vi "BMU参数读取-Auto.vi"(7 "Socket":dbl, 8 "CAN端口":u16(ring), 9 "设备索引号":u16(ring), 10 "CAN卡类型":u32(ring)=21, 11 "从板号":u8=1) -> (3 "成功?":bool)   [LabVIEW 2013] (continued)
                  n499 = local read "设备索引号"() -> (w673:u16)
                  n500 = local read "CAN卡类型"() -> (w674:u32)
                  n501 = Increment(x=w670) -> (x+1=w667:dbl)
                  n502 = local read "CAN端口"() -> (w672:u16)
                  n503 = Reshape Array(w671, w667) -> (w669:dbl[])
                  n504 = stacked-sequence {
                    tunnel: w674 -> [_ w682]
                    tunnel: w673 -> [_ w681]
                    tunnel: w672 -> [_ w680]
                    tunnel: w669 -> [_ w679]
                    tunnel: w668 -> [_ w678]
                    tunnel: w666 -> [_ w677]
                    tunnel: w665 -> [_ w676]
                    frame #0 {
                    }
                    frame #1 {
                      n505 = call "多帧发送机制(EV05).vi"("can卡类型"=w682, "设备索引号"=w681, "CAN端口"=w680, "命令"=w676, "板号"=w678, "命令序号"=w677, "输入数据"=w679) -> ("错误输出"=w675:errorcluster)  [unwired: 2 in, 10 out]
                      n506 = call <vilib>:"Clear Errors.vi"("error in (no error)"=w675) -> ()  [unwired: 6 in, 1 out]
                    }
                  }
                }
                frame #3 {
                  n507 = while {
                    tunnel: [w685] -> w683
                    i -> [w690]
                    stop <- w687 stop-if-true
                    n508 = local read "强制终止读写标记"() -> (w684:bool)
                    n509 = global read "EV05全局变量1.vi" "读取超时"() -> (w685:bool)
                    n510 = Greater Or Equal?(x=w690, y=30) -> (x >= y?=w688:bool)
                    n511 = Wait Until Next ms Multiple(millisecond multiple=u32 100 ("毫秒倍数")) -> ()  [unwired: 1 out]
                    n512 = Compound Arithmetic op=OR(w684, w685, w688) -> (w687:bool)
                  }
                }
                frame #4 {
                  n513 = call <vilib>:"Unset Busy.vi"() -> ()  [unwired: 2 in, 10 out]
                  n514 = case shown="假" w692 {
                    tunnel: w691 -> [w693 _]
                    frame False {
                      n515 = control-ref of="结果"() -> (w697:refnum<vi>)
                      n516 = Concatenate Strings(w693, "       写入失败" ("字符串")) -> (w696:string)
                      n517 = Build Array(w696) -> (w695:string[])
                      n518 = call "表格编辑.vi"("新元素/子数组"=w695, "活动单元格:单元格背景色"=u32 16740749, "MCListbox引用句柄"=w697) -> ()  [unwired: 9 out]
                    }
                    frame True {
                    }
                  }
                }
                frame #5 {
                  n519 = Increment(x=w703) -> (x+1=w699:i32)
                  n520 = Equal?(x=w704, y=w699) -> (x = y?=w702:bool)
                  n521 = And(x=w701, y=w702) -> (x .and. y?=w700:bool)
                  n522 = case shown="真" w700 {
                    frame False {
                    }
                    frame True {
                      n523 = control-ref of="结果"() -> (w708:refnum<vi>)
                      n524 = Concatenate Strings("写入完成" ("字符串")) -> (w707:string)
                      n525 = Build Array(w707) -> (w706:string[])
                      n526 = call "表格编辑.vi"("新元素/子数组"=w706, "活动单元格:单元格背景色"=u32 21937, "MCListbox引用句柄"=w708) -> ()  [unwired: 9 out]
                    }
                  }
                }
              }
            }
            n527 = local read "强制终止读写标记"() -> (w601:bool)
            n528 = Or(x=w599, y=w601) -> (x .or. y?=w600:bool)
          }
          n529 = stacked-sequence {
            tunnel: w591 -> [_]
            frame #0 {
              n530 = call <vilib>:"Unset Busy.vi"() -> ()  [unwired: 2 in, 10 out]
              n531 = local write "强制终止读写标记"(FALSE ("强制停止")) -> ()
            }
          }
        }
        frame "单个读取" {
          n532 = stacked-sequence {
            tunnel: [w741] -> w739
            frame #0 {
              n533 = local read "主从选择"() -> (w742:enum32{"主板", "从板"})
              n534 = case shown="\"主板\", 默认" w742 {
                tunnel: [w755 w838] -> w744
                tunnel: [w754 w839] -> w749
                tunnel: [0 ("从板号") w835] -> w748
                tunnel: [0 ("板号") u8 0 ("板号")] -> w747
                tunnel: [w750 w834] -> w745
                frame "主板", Default {
                  n535 = local read "主板选项"() -> (w751:string)
                  n536 = case shown="\"二维码\"" w751 {
                    tunnel: [_ u8[] [1, 2, 3, 4, 5, 6, 13, 8, 7, 9, 10, 11, 12] u8[] [1] u8[] [1] u8[] [1] u8[] [2] u8[] [3] u8[] [4] u8[] [5] u8[] [6] u8[] [13] u8[] [7] u8[] [8] u8[] [9] u8[] [10] u8[] [14] u8[] [11] u8[] [12] u8[] [2] u8[] [3] u8[] [1] u8[] [2] u8[] [1] u8[] [2] u8[] [3] u8[] [4] u8[] [1, 2, 3, 4]] -> w755
                    tunnel: [_ u8 128 ("命令") u8 129 ("命令") u8 128 ("命令") u8 140 ("命令") u8 128 ("命令") u8 128 ("命令") u8 128 ("命令") u8 128 ("命令") u8 128 ("命令") u8 128 ("命令") u8 128 ("命令") u8 128 ("命令") u8 128 ("命令") u8 128 ("命令") u8 128 ("命令") u8 128 ("命令") u8 128 ("命令") u8 129 ("命令") u8 129 ("命令") u8 130 ("命令") u8 130 ("命令") u8 132 ("命令") u8 132 ("命令") u8 132 ("命令") u8 132 ("命令") u8 132 ("命令")] -> w754
                    tunnel: [_ string[] ["产品编号", "电压个数", "通道电压数", "电压起始值", "温度个数", "温度起始值", "保险位置", "电池额定实际容量", "SOC", "配置文件版本", "参数修改记录", "车牌号", "SOH"] string[] ["一级故障阀值"] string[] ["产品编号"] string[] ["读二维码"] string[] ["电压个数"] string[] ["通道电压数"] string[] ["电压起始值"] string[] ["温度个数"] string[] ["温度起始值"] string[] ["保险位置"] string[] ["SOC"] string[] ["电池额定实际容量"] string[] ["配置文件版本"] string[] ["参数修改记录"] string[] ["校正时钟"] string[] ["车牌号"] string[] ["SOH"] string[] ["二级故障阀值"] string[] ["三级故障阀值"] string[] ["加热控制参数"] string[] ["充电控制参数"] string[] ["电池信息1"] string[] ["电池包组号"] string[] ["充放电安时"] string[] ["电池充放电次数"] string[] ["电池信息1", "电池包组号", "充放电安时", "电池充放电次数"]] -> w750
                    frame "假", Default {
                    }
                    frame "项目信息" {
                    }
                    frame "SOC过低", "SOC过高", "SOH过低", "充电电流过高", "单体电压过低", "单体电压过高", "单组电压不均衡", "单组温度不均衡", "放电电流过高", "极柱温度过高", "内阻过大", "温度过低", "温度过高", "一级故障阀值", "整组电压不均衡", "整组温度不均衡", "总电压过低", "总电压过高" {
                    }
                    frame "产品编号" {
                    }
                    frame "二维码" {
                    }
                    frame "电压个数" {
                    }
                    frame "通道电压数" {
                    }
                    frame "电压起始值" {
                    }
                    frame "温度个数" {
                    }
                    frame "温度起始值" {
                    }
                    frame "保险位置" {
                    }
                    frame "SOC" {
                    }
                    frame "电池额定实际容量" {
                    }
                    frame "配置文件版本" {
                    }
                    frame "参数修改记录" {
                    }
                    frame "校正时钟" {
                    }
                    frame "车牌号" {
                    }
                    frame "SOH" {
                    }
                    frame "SOC过低(2)", "SOC过高(2)", "SOH过低(2)", "充电电流过高(2)", "单体电压过低(2)", "单体电压过高(2)", "单组电压不均衡(2)", "单组温度不均衡(2)", "二级故障阀值", "放电电流过高(2)", "极柱温度过高(2)", "内阻过大(2)", "温度过低(2)", "温度过高(2)", "整组电压不均衡(2)", "整组温度不均衡(2)", "总电压过低(2)", "总电压过高(2)" {
                    }
                    frame "SOC过低(3)", "SOC过高(3)", "SOH过低(3)", "充电电流过高(3)", "单体电压过低(3)", "单体电压过高(3)", "单组电压不均衡(3)", "单组温度不均衡(3)", "放电电流过高(3)", "极柱温度过高(3)", "内阻过大(3)", "三级故障阀值", "温度过低(3)", "温度过高(3)", "整组电压不均衡(3)", "整组温度不均衡(3)", "总电压过低(3)", "总电压过高(3)" {
                    }
                    frame "风机关闭温差", "风机关闭温度", "风机开启温差", "风机开启温度", "加热关闭温差", "加热关闭温度", "加热开启温度", "加热控制参数" {
                    }
                    frame "充电控制参数", "电流步长", "最大允许充电电流", "最大允许充电温度", "最大允许单体电压", "最大允许总电压", "最小允许充电电流", "最小允许充电温度", "最小允许单体电压" {
                    }
                    frame "电池信息1" {
                    }
                    frame "电池包组号" {
                    }
                    frame "充放电安时" {
                    }
                    frame "电池充放电次数" {
                    }
                    frame "电池信息" {
                    }
                  }
                }
                frame "从板" {
                  n537 = local read "从板选项"() -> (w836:string)
                  n538 = case shown="\"二维码\"" w836 {
                    tunnel: [_ u8 0 ("命令") u8 10 ("命令") u8 0 ("命令") u8 0 ("命令") u8 0 ("命令") u8 0 ("命令") u8 0 ("命令") u8 0 ("命令") u8 2 ("命令") u8 2 ("命令") u8 2 ("命令") u8 3 ("命令") u8 6 ("命令") u8 6 ("命令") u8 6 ("命令") u8 3 ("命令") u8 3 ("命令") u8 3 ("命令") u8 3 ("命令") u8 3 ("命令") u8 3 ("命令") u8 3 ("命令")] -> w839
                    tunnel: [_ u8[] [6] u8[] [1] u8[] [6, 1, 2, 3, 4, 5] u8[] [1] u8[] [2] u8[] [3] u8[] [4] u8[] [5] u8[] [1] u8[] [2] u8[] [3] u8[] [1, 2, 3, 4, 5, 6, 7] u8[] [1, 2] u8[] [2] u8[] [1] u8[] [1] u8[] [2] u8[] [3] u8[] [4] u8[] [5] u8[] [6] u8[] [7]] -> w838
                    tunnel: [_ string[] ["从板号"] string[] ["读二维码"] string[] ["从板号", "电压起始值", "通道电压个数", "保险位置", "温度起始值", "加热控制参数"] string[] ["电压起始值"] string[] ["通道电压节数"] string[] ["保险位置"] string[] ["温度起始值"] string[] ["加热控制参数"] string[] ["一级故障阀值"] string[] ["二级故障阀值"] string[] ["三级故障阀值"] string[] ["电池包信息1", "电池包序号", "充放电安时", "充电次数时间", "SOC", "车牌号", "充电参数"] string[] ["均衡阀值", "充电结束电压"] string[] ["充电结束电压"] string[] ["均衡阀值"] string[] ["电池包信息1"] string[] ["电池包序号"] string[] ["充放电安时"] string[] ["充电次数时间"] string[] ["SOC"] string[] ["车牌号"] string[] ["充电参数"]] -> w834
                    frame "假", Default {
                    }
                    frame "从板号" {
                    }
                    frame "二维码" {
                    }
                    frame "从板信息" {
                    }
                    frame "电压个数" {
                    }
                    frame "通道电压节数" {
                    }
                    frame "保险位置" {
                    }
                    frame "温度个数" {
                    }
                    frame "风机关闭温差", "风机关闭温度", "风机开启温差", "风机开启温度", "加热关闭温差", "加热关闭温度", "加热开启温度", "加热控制参数" {
                    }
                    frame "SOC过低", "电压不均衡", "电压过低", "电压过高", "温度不均衡", "温度过低", "温度过高", "一级故障阀值" {
                    }
                    frame "SOC过低(2)", "电压不均衡(2)", "电压过低(2)", "电压过高(2)", "二级故障阀值", "温度不均衡(2)", "温度过低(2)", "温度过高(2)" {
                    }
                    frame "SOC过低(3)", "电压不均衡(3)", "电压过低(3)", "电压过高(3)", "三级故障阀值", "温度不均衡(3)", "温度过低(3)", "温度过高(3)" {
                    }
                    frame "快换参数" {
                    }
                    frame "均衡参数" {
                    }
                    frame "充电结束电压" {
                    }
                    frame "均衡阀值" {
                    }
                    frame "电池包信息1" {
                    }
                    frame "电池包序号" {
                    }
                    frame "充放电安时" {
                    }
                    frame "充电次数时间" {
                    }
                    frame "SOC" {
                    }
                    frame "车牌号" {
                    }
                    frame "充电参数" {
                    }
                  }
                  n539 = local read "从板号"() -> (w835:u8)
                }
              }
              n540 = Build Array(w747) -> (w746:i32[])
              n541 = local write "命令"(w749) -> ()
              n542 = Array Size(array=w744) -> (size(s)=w743:i32)
              n543 = for {
                tunnel: w744 -> [w914] mode=indexing
                tunnel: w749 -> [w913]
                tunnel: w748 -> [w912]
                tunnel: w746 -> [w911]
                tunnel: w745 -> [w910] mode=indexing
                tunnel: w743 -> [w909]
                tunnel: w742 -> [w907]
                tunnel: [w906] -> w741
                i -> [w908]
                n544 = while {
                  tunnel: w914 -> [w923]
                  tunnel: w913 -> [w922]
                  tunnel: w912 -> [w921]
                  tunnel: w911 -> [w920]
                  tunnel: w910 -> [w919]
                  tunnel: w909 -> [w918]
                  tunnel: w908 -> [w917]
                  tunnel: w907 -> [w916]
                  tunnel: [w915] -> w906
                  stop <- w915 stop-if-true
                  n545 = stacked-sequence {
                    seq-local: [_ _ _ _ w1073 _ _] -> [_ _ _ _ _ w1082 _]
                    tunnel: w923 -> [_ _ _ w1061 _ _ _]
                    tunnel: w922 -> [_ _ _ w1060 _ _ _]
                    tunnel: w921 -> [_ _ _ w1059 _ _ _]
                    tunnel: w920 -> [_ _ _ w1058 _ _ _]
                    tunnel: [_ _ _ _ w1074 _ _] -> w915
                    tunnel: w919 -> [w925 _ _ _ _ w1083 _]
                    tunnel: w918 -> [_ _ _ _ _ _ w1093]
                    tunnel: w917 -> [_ _ _ _ _ _ w1092]
                    tunnel: w916 -> [w924 _ _ _ _ _ _]
                    frame #0 {
                      n546 = case shown="\"从板\"" w924 {
                        tunnel: w925 -> [w926 w1018]
                        frame "主板", Default {
                          n547 = case shown="\"读二维码\"" w926 {
                            frame "假", Default {
                            }
                            frame "产品编号" {
                              n548 = control-ref of="产品编号"() -> (w928:refnum<vi>)
                              n549 = property class="Str"(reference=w928, "Value"="") -> ()  [unwired: 1 in, 2 out]
                            }
                            frame "读二维码" {
                              n550 = local write "二维码信息"("" ("二维码信息")) -> ()
                            }
                            frame "电压个数" {
                              n551 = local read "从板个数"() -> (w930:dbl)
                              n552 = control-ref of="项目信息"() -> (w934:refnum<vi>)
                              n553 = for {
                                N: w930 -> [_]
                                tunnel: [""] -> w933 mode=indexing
                              }
                              n554 = call "表格数据输入-8.6.vi"("行数"=u32 0, "列数"=u32 1, "字符串数组"=w933, "表格引用"=w934) -> ()  [unwired: 8 in]
                            }
                            frame "通道电压数" {
                              n555 = control-ref of="项目信息"() -> (w940:refnum<vi>)
                              n556 = for {
                                N: 20 -> [_]
                                tunnel: [""] -> w939 mode=indexing
                              }
                              n557 = local read "从板个数"() -> (w941:dbl)
                              n558 = Increment(x=w941) -> (x+1=w937:dbl)
                              n559 = call "表格数据输入-8.6.vi"("行数"=w937, "列数"=u32 1, "字符串数组"=w939, "表格引用"=w940) -> ()  [unwired: 8 in]
                            }
                            frame "电压起始值" {
                              n560 = local read "从板个数"() -> (w945:dbl)
                              n561 = Increment(x=w945) -> (x+1=w944:dbl)
                              n562 = control-ref of="项目信息"() -> (w951:refnum<vi>)
                              n563 = for {
                                N: w944 -> [_]
                                tunnel: [""] -> w950 mode=indexing
                              }
                              n564 = Multiply(x=u8 1, y=w945) -> (x*y=w947:dbl)
                              n565 = Add(x=w947, y=u8 21) -> (x+y=w943:dbl)
                              n566 = call "表格数据输入-8.6.vi"("行数"=w943, "列数"=u32 1, "字符串数组"=w950, "表格引用"=w951) -> ()  [unwired: 8 in]
                            }
                            frame "温度个数" {
                              n567 = local read "从板个数"() -> (w955:dbl)
                              n568 = Increment(x=w955) -> (x+1=w954:dbl)
                              n569 = control-ref of="项目信息"() -> (w961:refnum<vi>)
                              n570 = for {
                                N: w954 -> [_]
                                tunnel: [""] -> w960 mode=indexing
                              }
                              n571 = Multiply(x=u8 2, y=w955) -> (x*y=w957:dbl)
                              n572 = Add(x=w957, y=u8 22) -> (x+y=w953:dbl)
                              n573 = call "表格数据输入-8.6.vi"("行数"=w953, "列数"=u32 1, "字符串数组"=w960, "表格引用"=w961) -> ()  [unwired: 8 in]
                            }
                            frame "温度起始值" {
                              n574 = local read "从板个数"() -> (w965:dbl)
                              n575 = Increment(x=w965) -> (x+1=w964:dbl)
                              n576 = control-ref of="项目信息"() -> (w971:refnum<vi>)
                              n577 = for {
                                N: w964 -> [_]
                                tunnel: [""] -> w970 mode=indexing
                              }
                              n578 = Multiply(x=u8 3, y=w965) -> (x*y=w967:dbl)
                              n579 = Add(x=w967, y=u8 23) -> (x+y=w963:dbl)
                              n580 = call "表格数据输入-8.6.vi"("行数"=w963, "列数"=u32 1, "字符串数组"=w970, "表格引用"=w971) -> ()  [unwired: 8 in]
                            }
                            frame "保险位置" {
                              n581 = local read "从板个数"() -> (w975:dbl)
                              n582 = control-ref of="项目信息"() -> (w981:refnum<vi>)
                              n583 = for {
                                N: 10 -> [_]
                                tunnel: [""] -> w980 mode=indexing
                              }
                              n584 = Multiply(x=u8 4, y=w975) -> (x*y=w977:dbl)
                              n585 = Add(x=w977, y=u8 24) -> (x+y=w974:dbl)
                              n586 = call "表格数据输入-8.6.vi"("行数"=w974, "列数"=u32 1, "字符串数组"=w980, "表格引用"=w981) -> ()  [unwired: 8 in]
                            }
                            frame "电池额定实际容量" {
                              w983 = 0.0 ("值")
                              n587 = control-ref of="电池实际容量(A)"() -> (w984:refnum<vi>)
                              n588 = control-ref of="电池额定容量(A)"() -> (w985:refnum<vi>)
                              n589 = property class="DigNum (严格)"(reference=w984, "Value"=w983) -> ()  [unwired: 1 in, 2 out]
                              n590 = property class="DigNum (严格)"(reference=w985, "Value"=w983) -> ()  [unwired: 1 in, 2 out]
                            }
                            frame "SOC" {
                              n591 = control-ref of="SOC(%)"() -> (w986:refnum<vi>)
                              n592 = property class="DigNum (严格)"(reference=w986, "Value"=0.0 ("值")) -> ()  [unwired: 1 in, 2 out]
                            }
                            frame "配置文件版本" {
                              n593 = control-ref of="配置文件版本"() -> (w988:refnum<vi>)
                              n594 = property class="Str"(reference=w988, "Value"="" ("值")) -> ()  [unwired: 1 in, 2 out]
                            }
                            frame "参数修改记录" {
                              n595 = control-ref of="使用者"() -> (w991:refnum<vi>)
                              n596 = control-ref of="系统时钟"() -> (w992:refnum<vi>)
                              n597 = property class="DigNum (严格)"(reference=w991, "Value"=0.0 ("值")) -> ()  [unwired: 1 in, 2 out]
                              n598 = property class="Str"(reference=w992, "Value"="" ("值")) -> ()  [unwired: 1 in, 2 out]
                            }
                            frame "校正时钟" {
                              n599 = control-ref of="系统时钟"() -> (w994:refnum<vi>)
                              n600 = property class="Str"(reference=w994, "Value"="" ("值")) -> ()  [unwired: 1 in, 2 out]
                            }
                            frame "车牌号" {
                              n601 = control-ref of="车架(牌)号"() -> (w996:refnum<vi>)
                              n602 = property class="Str"(reference=w996, "Value"="" ("值")) -> ()  [unwired: 1 in, 2 out]
                            }
                            frame "SOH" {
                              n603 = control-ref of="SOH(%)"() -> (w999:refnum<vi>)
                              n604 = property class="DigNum (严格)"(reference=w999, "Value"=0.0 ("值")) -> ()  [unwired: 1 in, 2 out]
                            }
                            frame "一级故障阀值" {
                              n605 = local write "一级故障"(T11 {"总电压过高"=0.0, "整组电压不均衡"=0.0, "SOC过高"=0.0, "单体电压过高"=0.0, "总电压过低"=0.0, "温度过高"=0.0, "温度过低"=0.0, "单组电压不均衡"=0.0, "整组温度不均衡"=0.0, "单组温度不均衡"=0.0, "单体电压过低"=0.0, "充电电流过高"=0.0, "放电电流过高"=0.0, "SOC过低"=0.0, "内阻过大"=0.0, "极柱温度过高"=0.0, "SOH过低"=0.0} ("一级故障")) -> ()
                            }
                            frame "二级故障阀值" {
                              n606 = local write "一级故障 2"(T11 {"总电压过高"=0.0, "整组电压不均衡"=0.0, "SOC过高"=0.0, "单体电压过高"=0.0, "总电压过低"=0.0, "温度过高"=0.0, "温度过低"=0.0, "单组电压不均衡"=0.0, "整组温度不均衡"=0.0, "单组温度不均衡"=0.0, "单体电压过低"=0.0, "充电电流过高"=0.0, "放电电流过高"=0.0, "SOC过低"=0.0, "内阻过大"=0.0, "极柱温度过高"=0.0, "SOH过低"=0.0} ("一级故障")) -> ()
                            }
                            frame "三级故障阀值" {
                              n607 = local write "一级故障 3"(T11 {"总电压过高"=0.0, "整组电压不均衡"=0.0, "SOC过高"=0.0, "单体电压过高"=0.0, "总电压过低"=0.0, "温度过高"=0.0, "温度过低"=0.0, "单组电压不均衡"=0.0, "整组温度不均衡"=0.0, "单组温度不均衡"=0.0, "单体电压过低"=0.0, "充电电流过高"=0.0, "放电电流过高"=0.0, "SOC过低"=0.0, "内阻过大"=0.0, "极柱温度过高"=0.0, "SOH过低"=0.0} ("一级故障")) -> ()
                            }
                            frame "加热控制参数" {
                              n608 = local write "加热控制参数"(T12 {"风机开启温度"=0.0, "风机关闭温度"=0.0, "加热开启温度"=0.0, "加热关闭温度"=0.0, "风机开启温差"=0.0, "风机关闭温差"=0.0, "加热关闭温差"=0.0} ("加热控制参数")) -> ()
                            }
                            frame "充电控制参数" {
                              n609 = local write "一级故障 5"(T13 {"最大允许单体电压"=0.0, "最大允许总电压"=0.0, "最小允许单体电压"=0.0, "最大允许充电电流"=0.0, "最小允许充电电流"=0.0, "最大允许充电温度"=0.0, "最小允许充电温度"=0.0, "电流步长"=0.0} ("一级故障 5")) -> ()
                            }
                            frame "电池信息1" {
                              w1005 = ""
                              w1006 = 0.0 ("电池串联")
                              n610 = local read "电池信息"() -> (w1008:T14)
                              n611 = Bundle By Name(cluster=w1008, "电池串联"=w1006, "电池并联"=w1006, "电池包额定容量"=w1006, "电池包额定能量(kWh)"=w1006, "电池包额定总电压"=w1006, "实际容量"=w1006, "电池厂家"=w1005, "电池类型"=w1005, "电池生产日期"=w1005) -> (w1007:T14)
                              n612 = local write "电池信息"(w1007) -> ()
                            }
                            frame "电池包组号" {
                              n613 = local read "电池信息"() -> (w1011:T14)
                              n614 = Bundle By Name(cluster=w1011, "电池包组号"="") -> (w1010:T14)
                              n615 = local write "电池信息"(w1010) -> ()
                            }
                            frame "充放电安时" {
                              w1012 = 0.0 ("累计充电总安时")
                              n616 = local read "电池信息"() -> (w1014:T14)
                              n617 = Bundle By Name(cluster=w1014, "累计充电总安时"=w1012, "累计放电总安时"=w1012) -> (w1013:T14)
                              n618 = local write "电池信息"(w1013) -> ()
                            }
                            frame "电池充放电次数" {
                              w1015 = 0.0 ("累计充电总安时")
                              n619 = local read "电池信息"() -> (w1017:T14)
                              n620 = Bundle By Name(cluster=w1017, "电池充满次数"=w1015, "电池放空次数"=w1015, "电池充电次数"=w1015) -> (w1016:T14)
                              n621 = local write "电池信息"(w1016) -> ()
                            }
                          }
                        }
                        frame "从板" {
                          n622 = case shown="\"读二维码\"" w1018 {
                            frame "假", Default {
                            }
                            frame "电压起始值" {
                              n623 = control-ref of="项目信息 2"() -> (w1020:refnum<vi>)
                              n624 = for {
                                N: 1 -> [_]
                                tunnel: [""] -> w1023 mode=indexing
                              }
                              n625 = call "表格数据输入-8.6.vi"("行数"=u32 0, "列数"=u32 1, "字符串数组"=w1023, "表格引用"=w1020) -> ()  [unwired: 8 in]
                            }
                            frame "读二维码" {
                              n626 = local write "二维码信息 2"("" ("二维码信息 2")) -> ()
                            }
                            frame "通道电压节数" {
                              n627 = control-ref of="项目信息 2"() -> (w1026:refnum<vi>)
                              n628 = for {
                                N: 5 -> [_]
                                tunnel: [""] -> w1030 mode=indexing
                              }
                              n629 = call "表格数据输入-8.6.vi"("行数"=u32 22, "列数"=u32 1, "字符串数组"=w1030, "表格引用"=w1026) -> ()  [unwired: 8 in]
                            }
                            frame "保险位置" {
                              n630 = control-ref of="项目信息 2"() -> (w1032:refnum<vi>)
                              n631 = for {
                                N: 20 -> [_]
                                tunnel: [""] -> w1036 mode=indexing
                              }
                              n632 = call "表格数据输入-8.6.vi"("行数"=u32 2, "列数"=u32 1, "字符串数组"=w1036, "表格引用"=w1032) -> ()  [unwired: 8 in]
                            }
                            frame "温度起始值" {
                              n633 = control-ref of="项目信息 2"() -> (w1038:refnum<vi>)
                              n634 = for {
                                N: 1 -> [_]
                                tunnel: [""] -> w1042 mode=indexing
                              }
                              n635 = call "表格数据输入-8.6.vi"("行数"=u32 1, "列数"=u32 1, "字符串数组"=w1042, "表格引用"=w1038) -> ()  [unwired: 8 in]
                            }
                            frame "加热控制参数" {
                              n636 = local write "加热控制参数"(T12 {"风机开启温度"=0.0, "风机关闭温度"=0.0, "加热开启温度"=0.0, "加热关闭温度"=0.0, "风机开启温差"=0.0, "风机关闭温差"=0.0, "加热关闭温差"=0.0} ("加热控制参数")) -> ()
                            }
                            frame "一级故障阀值" {
                              n637 = local write "一级故障 6"(T16 {"电压过高"=0.0, "电压过低"=0.0, "温度过高"=0.0, "温度过低"=0.0, "电压不均衡(V)"=0.0, "温度不均衡"=0.0, "SOC过低"=0.0} ("一级故障 6")) -> ()
                            }
                            frame "二级故障阀值" {
                              n638 = local write "一级故障 7"(T16 {"电压过高"=0.0, "电压过低"=0.0, "温度过高"=0.0, "温度过低"=0.0, "电压不均衡(V)"=0.0, "温度不均衡"=0.0, "SOC过低"=0.0} ("一级故障 7")) -> ()
                            }
                            frame "三级故障阀值" {
                              n639 = local write "一级故障 8"(T16 {"电压过高"=0.0, "电压过低"=0.0, "温度过高"=0.0, "温度过低"=0.0, "电压不均衡(V)"=0.0, "温度不均衡"=0.0, "SOC过低"=0.0} ("一级故障 7")) -> ()
                            }
                            frame "均衡参数" {
                              n640 = local write "均衡参数"(T18 {"充电结束电压(90%)"=0.0, "充电结束电压(91%)"=0.0, "充电结束电压(92%)"=0.0, "充电结束电压(93%)"=0.0, "充电结束电压(94%)"=0.0, "均衡计算-电压高阀值1级"=0.0, "均衡计算-电压高阀值2级"=0.0, "均衡计算-电压低阀值1级"=0.0, "均衡计算-电压低阀值2级"=0.0, "均衡计算-最低电压阀值"=0.0, "均衡停止-最低电压阀值"=0.0, "均衡计算-电压极差阀值"=0.0, "充电结束电压(95%)"=0.0, "充电结束电压(96%)"=0.0, "充电结束电压(97%)"=0.0, "充电结束电压(98%)"=0.0, "充电结束电压(99%)"=0.0, "充电结束电压(100%)"=0.0} ("均衡参数")) -> ()
                            }
                            frame "均衡阀值" {
                              w1049 = sgl 0.0 ("均衡计算-电压高阀值1级")
                              n641 = local read "均衡参数"() -> (w1050:T18)
                              n642 = Bundle By Name(cluster=w1050, "均衡计算-电压高阀值1级"=w1049, "均衡计算-电压高阀值2级"=w1049, "均衡计算-电压低阀值1级"=w1049, "均衡计算-电压低阀值2级"=w1049, "均衡计算-最低电压阀值"=w1049, "均衡停止-最低电压阀值"=w1049, "均衡计算-电压极差阀值"=w1049) -> (w1051:T18)
                              n643 = local write "均衡参数"(w1051) -> ()
                            }
                            frame "充电结束电压" {
                              w1052 = sgl 0.0 ("均衡计算-电压高阀值1级")
                              n644 = local read "均衡参数"() -> (w1053:T18)
                              n645 = Bundle By Name(cluster=w1053, "充电结束电压(90%)"=w1052, "充电结束电压(91%)"=w1052, "充电结束电压(92%)"=w1052, "充电结束电压(93%)"=w1052, "充电结束电压(94%)"=w1052, "充电结束电压(95%)"=w1052, "充电结束电压(96%)"=w1052, "充电结束电压(97%)"=w1052, "充电结束电压(98%)"=w1052, "充电结束电压(99%)"=w1052, "充电结束电压(100%)"=w1052) -> (w1054:T18)
                              n646 = local write "均衡参数"(w1054) -> ()
                            }
                          }
                        }
                      }
                    }
                    frame #1 {
                      w1055 = FALSE ("流控帧")
                      w1056 = TRUE ("流控帧 2")
                      n647 = global write "EV05全局变量1.vi" "写入超时"(w1055) -> ()
                      n648 = global write "EV05全局变量1.vi" "流控帧"(w1055) -> ()
                      n649 = local write "写?"(w1055) -> ()
                      n650 = call <vilib>:"Set Busy.vi"("disable click? (T)"=w1055) -> ()  [unwired: 3 in, 8 out]
                      n651 = local write "消除"(w1056) -> ()
                      n652 = local write "控制1"(w1056) -> ()
                      n653 = global write "EV05全局变量1.vi" "流控帧 2"(w1056) -> ()
                    }
                    frame #2 {
                      n654 = Wait Until Next ms Multiple(millisecond multiple=u32 150 ("毫秒倍数")) -> ()  [unwired: 1 out]
                    }
                    frame #3 {
                      n655 = local read "设备索引号"() -> (w1063:u16)
                      n656 = local read "CAN卡类型"() -> (w1064:u32)
                      n657 = local read "CAN端口"() -> (w1062:u16)
                      n658 = stacked-sequence {
                        tunnel: w1064 -> [_ w1072]
                        tunnel: w1063 -> [_ w1071]
                        tunnel: w1062 -> [_ w1070]
                        tunnel: w1061 -> [_ w1069]
                        tunnel: w1060 -> [_ w1068]
                        tunnel: w1059 -> [_ w1067]
                        tunnel: w1058 -> [_ w1066]
                        frame #0 {
                        }
                        frame #1 {
                          n659 = call "多帧发送机制(EV05).vi"("can卡类型"=w1072, "设备索引号"=w1071, "CAN端口"=w1070, "命令"=w1068, "板号"=w1067, "命令序号"=w1069, "输入数据"=w1066) -> ("错误输出"=w1065:errorcluster)  [unwired: 2 in, 10 out]
                          n660 = call <vilib>:"Clear Errors.vi"("error in (no error)"=w1065) -> ()  [unwired: 6 in, 1 out]
                        }
                      }
                      "命令序号" <- w1061
                    }
                    frame #4 {
                      n661 = while {
                        tunnel: [w1077] -> w1074
                        tunnel: [w1076] -> w1073
                        i -> [w1080]
                        stop <- w1077 stop-if-true
                        n662 = local read "强制终止读写标记"() -> (w1075:bool)
                        n663 = global read "EV05全局变量1.vi" "写入超时"() -> (w1076:bool)
                        n664 = Greater Or Equal?(x=w1080, y=30) -> (x >= y?=w1078:bool)
                        n665 = Compound Arithmetic op=OR(w1075, w1076, w1078) -> (w1077:bool)
                        n666 = Wait Until Next ms Multiple(millisecond multiple=u32 100 ("毫秒倍数")) -> ()  [unwired: 1 out]
                      }
                    }
                    frame #5 {
                      n667 = case shown="假" w1082 {
                        tunnel: w1083 -> [w1086 _]
                        frame False {
                          n668 = control-ref of="结果"() -> (w1085:refnum<vi>)
                          n669 = Concatenate Strings(w1086, "     读取失败" ("字符串")) -> (w1088:string)
                          n670 = Build Array(w1088) -> (w1084:string[])
                          n671 = call "表格编辑.vi"("新元素/子数组"=w1084, "活动单元格:单元格背景色"=u32 16740749, "MCListbox引用句柄"=w1085) -> ()  [unwired: 9 out]
                        }
                        frame True {
                        }
                      }
                    }
                    frame #6 {
                      n672 = Increment(x=w1092) -> (x+1=w1091:i32)
                      n673 = Equal?(x=w1093, y=w1091) -> (x = y?=w1090:bool)
                      n674 = case shown="真" w1090 {
                        frame False {
                        }
                        frame True {
                          n675 = control-ref of="结果"() -> (w1095:refnum<vi>)
                          n676 = Concatenate Strings("读取完成" ("字符串")) -> (w1097:string)
                          n677 = Build Array(w1097) -> (w1094:string[])
                          n678 = call "表格编辑.vi"("新元素/子数组"=w1094, "活动单元格:单元格背景色"=u32 21937, "MCListbox引用句柄"=w1095) -> ()  [unwired: 9 out]
                        }
                      }
                    }
                  }
                }
              }
            }
          }
          n679 = stacked-sequence {
            tunnel: w739 -> [_]
            frame #0 {
              n680 = call <vilib>:"Unset Busy.vi"() -> ()  [unwired: 11 in, 1 out]
              n681 = local write "强制终止读写标记"(FALSE ("强制停止")) -> ()
            }
          }
        }
        frame "全部读取" {
          n682 = stacked-sequence {
            seq-local: [w1104 _ _ _] -> [_ _ _ w2100]
            seq-local: [w1103 _ _ _] -> [_ _ _ _]
            tunnel: [_ _ w1729 _] -> w1101
            tunnel: w1099 -> [_ w1300 _ _]
            frame #0 {
              n683 = local read "主从选择"() -> (w1104:enum32{"主板", "从板"})
              n684 = local read "路径"() -> (w1105:path)
              n685 = Empty String/Path?(string/path=w1105) -> (empty?=w1103:bool)
              n686 = disable-structure shown="禁用" {
                disable-tunnel: w1105 -> [w1108 _]
                disable-tunnel: w1103 -> [w1107 _]
                disable-tunnel: w1104 -> [w1106 _]
                frame Disabled {
                  n687 = case shown="假" w1107 {
                    tunnel: w1108 -> [w1112 _]
                    tunnel: w1106 -> [w1111 _]
                    frame False {
                      n688 = control-ref of="结果"() -> (w1109:refnum<vi>)
                      n689 = call-poly <vilib>:"Read From Spreadsheet File.vi"("file path (dialog if empty)"=w1112) -> ("all rows"=w1110:string[][])  [unwired: 3 in, 7 out]
                      n690 = case shown="\"主板\", 默认" w1111 {
                        tunnel: w1110 -> [w1114 w1209]
                        tunnel: w1109 -> [w1113 w1208]
                        frame "主板", Default {
                          n691 = stacked-sequence {
                            tunnel: w1114 -> [w1123 w1147 w1204]
                            tunnel: w1113 -> [w1120 _ w1175]
                            frame #0 {
                              n692 = Index Array(array=w1123, index (col)=3 ("禁用的索引 (列)")) -> (element=w1137:string[])  [unwired: 1 in]
                              n693 = Index Array(array=w1123, index (col)=1 ("禁用的索引 (列)")) -> (element=w1143:string[])  [unwired: 1 in]
                              n694 = Delete From Array(array=w1137, length=4 ("长度"), index=0 ("索引")) -> (deleted portion=w1134:string[], array with subset deleted=w1128:string[])
                              n695 = Delete From Array(array=w1143, length=1 ("长度"), index=0 ("索引")) -> (deleted portion=w1140:string[], array with subset deleted=w1117:string[])
                              n696 = Build Array("正在读取主板配置文件...") -> (w1121:string[])
                              n697 = Index Array(array=w1128) -> (element #1=w1127:string, element #2=w1126:string, element #3=w1125:string, element #4=w1124:string)  [unwired: 4 in]
                              n698 = for {
                                tunnel: w1134 -> [w1146] mode=indexing
                                tunnel: [w1145] -> w1133 mode=indexing
                                n699 = Fract/Exp String To Number(string=w1146) -> (number=w1145:dbl)  [unwired: 4 out]
                              }
                              n700 = Index Array(array=w1140) -> (element=w1139:string)  [unwired: 1 in]
                              n701 = global write "读配置文件全局.vi" "表格输入"(w1117) -> ()
                              n702 = call "表格编辑.vi"("新元素/子数组"=w1121, "活动单元格:单元格背景色"=u32 6618880, "MCListbox引用句柄"=w1120) -> ()  [unwired: 9 out]
                              n703 = Decimal String To Number(string=w1139) -> (number=w1118:i32)  [unwired: 1 in, 2 out]
                              n704 = global read "读配置文件全局.vi" "项目信息"() -> (w1116:T23)
                              n705 = Index Array(array=w1133) -> (element #1=w1132:dbl, element #2=w1131:dbl, element #3=w1130:dbl, element #4=w1129:dbl)  [unwired: 4 in]
                              n706 = global write "读配置文件全局.vi" "从板个数"(w1118) -> ()
                              n707 = Bundle(cluster=w1116, "电池额定容量"=w1132, "电池实际容量"=w1131, "车牌号"=w1127, "配置文件版本"=w1126, "SOH"=w1129, "SOC"=w1130, "产品编号"=w1125, "系统时钟"=w1124) -> (w1115:T23)  [unwired: 1 out]
                              n708 = global write "读配置文件全局.vi" "项目信息"(w1115) -> ()
                            }
                            frame #1 {
                              n709 = Index Array(array=w1147, index (col)=3 ("禁用的索引 (列)")) -> (element=w1165:string[])  [unwired: 1 in]
                              n710 = Index Array(array=w1147, index (col)=5 ("禁用的索引 (列)")) -> (element=w1159:string[])  [unwired: 1 in]
                              n711 = for {
                                tunnel: w1159 -> [w1172] mode=indexing
                                tunnel: [w1171] -> w1158 mode=indexing
                                n712 = Fract/Exp String To Number(string=w1172) -> (number=w1171:dbl)  [unwired: 4 out]
                              }
                              n713 = Delete From Array(array=w1165, length=17 ("长度"), index=8 ("索引")) -> (deleted portion=w1163:string[])  [unwired: 1 out]
                              n714 = for {
                                tunnel: w1163 -> [w1174] mode=indexing
                                tunnel: [w1173] -> w1161 mode=indexing
                                n715 = Fract/Exp String To Number(string=w1174) -> (number=w1173:dbl)  [unwired: 4 out]
                              }
                              n716 = global write "读配置文件全局.vi" "二级故障"(w1158) -> ()
                              n717 = global write "读配置文件全局.vi" "一级故障"(w1161) -> ()
                              n718 = Index Array(array=w1147, index (col)=7 ("禁用的索引 (列)")) -> (element=w1156:string[])  [unwired: 1 in]
                              n719 = Index Array(array=w1147, index (col)=9 ("禁用的索引 (列)")) -> (element=w1153:string[])  [unwired: 1 in]
                              n720 = for {
                                tunnel: w1156 -> [w1170] mode=indexing
                                tunnel: [w1169] -> w1155 mode=indexing
                                n721 = Fract/Exp String To Number(string=w1170) -> (number=w1169:dbl)  [unwired: 4 out]
                              }
                              n722 = for {
                                tunnel: w1153 -> [w1168] mode=indexing
                                tunnel: [w1167] -> w1152 mode=indexing
                                n723 = Fract/Exp String To Number(string=w1168) -> (number=w1167:dbl)  [unwired: 4 out]
                              }
                              n724 = Delete From Array(array=w1152, length=6 ("长度"), index=0 ("索引")) -> (deleted portion=w1149:dbl[], array with subset deleted=w1148:dbl[])
                              n725 = global write "读配置文件全局.vi" "三级故障"(w1155) -> ()
                              n726 = global write "读配置文件全局.vi" "加热控制参数"(w1149) -> ()
                              n727 = global write "读配置文件全局.vi" "充电控制参数"(w1148) -> ()
                            }
                            frame #2 {
                              n728 = call <vilib>:"Unset Busy.vi"() -> ()  [unwired: 2 in, 10 out]
                              n729 = Index Array(array=w1204, index (col)=11 ("禁用的索引 (列)")) -> (element=w1201:string[])  [unwired: 1 in]
                              n730 = Delete From Array(array=w1201, length=6 ("长度"), index=0 ("索引")) -> (deleted portion=w1183:string[], array with subset deleted=w1182:string[])
                              n731 = for {
                                tunnel: w1182 -> [w1207] mode=indexing
                                tunnel: [w1206] -> w1200 mode=indexing
                                n732 = Fract/Exp String To Number(string=w1207) -> (number=w1206:dbl)  [unwired: 4 out]
                              }
                              n733 = Index Array(array=w1183) -> (element #1=w1199:string, element #2=w1198:string, element #3=w1197:string, element #4=w1196:string, element #5=w1195:string, element #6=w1194:string)  [unwired: 6 in]
                              n734 = Index Array(array=w1200) -> (element #1=w1193:dbl, element #2=w1192:dbl, element #3=w1191:dbl, element #4=w1190:dbl, element #5=w1189:dbl, element #6=w1188:dbl, element #7=w1187:dbl, element #8=w1186:dbl, element #9=w1185:dbl, element #10=w1184:dbl, element #11=w1179:dbl)  [unwired: 11 in]
                              n735 = global read "读配置文件全局.vi" "电池信息"() -> (w1181:T24)
                              n736 = Build Array("配置文件读取完成") -> (w1177:string[])
                              n737 = Bundle(cluster=w1181, "电池串联"=w1193, "电池并联"=w1192, "累计放电总安时"=w1190, "电池包额定容量"=w1189, "电池包额定能量"=w1188, "电池包额定总电压"=w1187, "累计充电总安时"=w1191, "电池充满次数"=w1186, "电池放空次数"=w1185, "电池充电次数"=w1184, "电池生产日期"=w1199, "电池厂家"=w1198, "电池类型"=w1197, "电池包组号"=w1196, "电池包产权标识"=w1195, "电池应用车型"=w1194, "实际容量"=w1179) -> (w1180:T24)
                              n738 = call "表格编辑.vi"("新元素/子数组"=w1177, "活动单元格:单元格背景色"=u32 6618880, "MCListbox引用句柄"=w1175) -> ()  [unwired: 9 out]
                              n739 = global write "读配置文件全局.vi" "电池信息"(w1180) -> ()
                            }
                          }
                        }
                        frame "从板" {
                          n740 = stacked-sequence {
                            tunnel: w1209 -> [w1217 w1245 w1289]
                            tunnel: w1208 -> [w1214 _ w1265]
                            frame #0 {
                              n741 = Index Array(array=w1217, index (col)=1 ("禁用的索引 (列)")) -> (element=w1227:string[])  [unwired: 1 in]
                              n742 = Index Array(array=w1217, index (col)=3 ("禁用的索引 (列)")) -> (element=w1221:string[])  [unwired: 1 in]
                              n743 = Delete From Array(array=w1227, length=1 ("长度"), index=0 ("索引")) -> (deleted portion=w1224:string[], array with subset deleted=w1211:string[])
                              n744 = Delete From Array(array=w1221, length=6 ("长度"), index=0 ("索引")) -> (deleted portion=w1218:string[])  [unwired: 1 out]
                              n745 = for {
                                tunnel: w1218 -> [w1230] mode=indexing
                                tunnel: [w1229] -> w1210 mode=indexing
                                i -> [w1231]
                                n746 = Fract/Exp String To Number(string=w1230, default (0 dbl)=w1231) -> (number=w1229:i32)  [unwired: 3 out]
                              }
                              n747 = Index Array(array=w1224) -> (element=w1223:string)  [unwired: 1 in]
                              n748 = global write "读配置文件全局2.vi" "表格"(w1211) -> ()
                              n749 = Build Array("正在读取从板配置文件...") -> (w1215:string[])
                              n750 = Decimal String To Number(string=w1223) -> (number=w1212:i32)  [unwired: 1 in, 2 out]
                              n751 = call "表格编辑.vi"("新元素/子数组"=w1215, "活动单元格:单元格背景色"=u32 6618880, "MCListbox引用句柄"=w1214) -> ()  [unwired: 9 out]
                              n752 = global write "读配置文件全局2.vi" "加热控制参数"(w1210) -> ()
                              n753 = global write "读配置文件全局2.vi" "从板板号"(w1212) -> ()
                            }
                            frame #1 {
                              n754 = Index Array(array=w1245, index (col)=3 ("禁用的索引 (列)")) -> (element=w1235:string[])  [unwired: 1 in]
                              n755 = Array Subset(array=w1235, index=6 ("索引"), length=7 ("长度")) -> (w1242:string[])
                              n756 = Array Subset(array=w1235, index=13 ("索引"), length=7 ("长度")) -> (w1241:string[])
                              n757 = Array Subset(array=w1235, index=20 ("索引"), length=7 ("长度")) -> (w1236:string[])
                              n758 = for {
                                tunnel: w1242 -> [w1252] mode=indexing
                                tunnel: [w1251] -> w1232 mode=indexing
                                n759 = Fract/Exp String To Number(string=w1252) -> (number=w1251:dbl)  [unwired: 4 out]
                              }
                              n760 = for {
                                tunnel: w1241 -> [w1250] mode=indexing
                                tunnel: [w1249] -> w1233 mode=indexing
                                n761 = Fract/Exp String To Number(string=w1250) -> (number=w1249:dbl)  [unwired: 4 out]
                              }
                              n762 = for {
                                tunnel: w1236 -> [w1248] mode=indexing
                                tunnel: [w1247] -> w1234 mode=indexing
                                n763 = Fract/Exp String To Number(string=w1248) -> (number=w1247:dbl)  [unwired: 4 out]
                              }
                              n764 = global write "读配置文件全局2.vi" "一级故障阀值"(w1232) -> ()
                              n765 = global write "读配置文件全局2.vi" "二级故障阀值"(w1233) -> ()
                              n766 = global write "读配置文件全局2.vi" "三级故障阀值"(w1234) -> ()
                            }
                            frame #2 {
                              n767 = Index Array(array=w1289, index (col)=5 ("禁用的索引 (列)")) -> (element=w1287:string[])  [unwired: 1 in]
                              n768 = Delete From Array(array=w1287, length=1 ("长度"), index=16 ("索引")) -> (deleted portion=w1283:string[], array with subset deleted=w1284:string[])
                              n769 = for {
                                tunnel: w1284 -> [w1292] mode=indexing
                                tunnel: [w1291] -> w1288 mode=indexing
                                n770 = Fract/Exp String To Number(string=w1292) -> (number=w1291:dbl)  [unwired: 4 out]
                              }
                              n771 = Index Array(array=w1288) -> (element #1=w1282:dbl, element #2=w1281:dbl, element #3=w1280:dbl, element #4=w1279:dbl, element #5=w1278:dbl, element #6=w1277:dbl, element #7=w1276:dbl, element #8=w1275:dbl, element #9=w1274:dbl, element #10=w1273:dbl, element #11=w1272:dbl, element #12=w1263:dbl, element #13=w1271:dbl, element #14=w1270:dbl, element #15=w1269:dbl, element #16=w1268:dbl, element #17=w1261:dbl, element #18=w1260:dbl, element #19=w1259:dbl, element #20=w1258:dbl, element #21=w1257:dbl, element #22=w1256:dbl)  [unwired: 22 in]
                              n772 = Build Array("配置文件读取完成") -> (w1266:string[])
                              n773 = Index Array(array=w1283, index=22 ("索引")) -> (element=w1262:string)
                              n774 = global read "读配置文件全局2.vi" "电池组信息"() -> (w1254:T25)
                              n775 = call "表格编辑.vi"("新元素/子数组"=w1266, "活动单元格:单元格背景色"=u32 6618880, "MCListbox引用句柄"=w1265) -> ()  [unwired: 9 out]
                              n776 = Bundle(cluster=w1254, "电池类型"=w1282, "电池厂家"=w1281, "电池地区"=w1280, "电池组序号"=w1279, "电池包串联数"=w1278, "电池包并联数"=w1277, "电池包安时数"=w1276, "电池包序号"=w1275, "充电次数"=w1274, "充满电时间"=w1273, "放空时间"=w1272, "车牌号"=w1262, "最大允许单体电压"=w1263, "最大允许总电压"=w1271, "最大允许温度"=w1270, "最小允许温度"=w1269, "最大允许充电电流"=w1268, "最小允许充电电流"=w1261, "最小允许单体电压"=w1260, "电流步长"=w1259, "SOC"=w1258, "充电总安时"=w1257, "放电总这时"=w1256) -> (w1253:T25)
                              n777 = call <vilib>:"Unset Busy.vi"() -> ()  [unwired: 2 in, 10 out]
                              n778 = global write "读配置文件全局2.vi" "电池组信息"(w1253) -> ()
                            }
                          }
                        }
                      }
                    }
                    frame True {
                    }
                  }
                }
                frame Enabled {
                }
              }
              n779 = case shown="\"从板\"" w1104 {
                frame "主板", Default {
                  w1293 = FALSE
                  n780 = global write "读配置文件全局.vi" "SOC判定"(w1293) -> ()
                  n781 = global write "读配置文件全局.vi" "SOH判定"(w1293) -> ()
                  n782 = global write "读配置文件全局.vi" "车牌号判定"(w1293) -> ()
                  n783 = global write "读配置文件全局.vi" "电池信息1判定"(w1293) -> ()
                  n784 = global write "读配置文件全局.vi" "保险位置判定"(w1293) -> ()
                  n785 = global write "读配置文件全局.vi" "产品编号判定"(w1293) -> ()
                  n786 = global write "读配置文件全局.vi" "充放电安时判定"(w1293) -> ()
                  n787 = global write "读配置文件全局.vi" "从板个数判定"(w1293) -> ()
                  n788 = global write "读配置文件全局.vi" "电池包组号判定"(w1293) -> ()
                  n789 = global write "读配置文件全局.vi" "电压个数判定"(w1293) -> ()
                  n790 = global write "读配置文件全局.vi" "电压起始值判定"(w1293) -> ()
                  n791 = global write "读配置文件全局.vi" "充电控制参数判定"(w1293) -> ()
                  n792 = global write "读配置文件全局.vi" "电池充放电次数判定"(w1293) -> ()
                  n793 = global write "读配置文件全局.vi" "电池额定实际容量判定"(w1293) -> ()
                  n794 = global write "读配置文件全局.vi" "二级故障判定"(w1293) -> ()
                  n795 = global write "读配置文件全局.vi" "三级故障判定"(w1293) -> ()
                  n796 = global write "读配置文件全局.vi" "通道电压数判定"(w1293) -> ()
                  n797 = global write "读配置文件全局.vi" "温度个数判定"(w1293) -> ()
                  n798 = global write "读配置文件全局.vi" "一级故障判定"(w1293) -> ()
                  n799 = global write "读配置文件全局.vi" "温度起始值判定"(w1293) -> ()
                  n800 = global write "读配置文件全局.vi" "加热控制参数判定"(w1293) -> ()
                  n801 = global write "读配置文件全局.vi" "配置文件版本判定"(w1293) -> ()
                }
                frame "从板" {
                  w1296 = FALSE
                  n802 = control-ref of="BMU读取结果"() -> (w1295:refnum<vi>)
                  n803 = global write "读配置文件全局2.vi" "从板号判定"(w1296) -> ()
                  n804 = global write "读配置文件全局2.vi" "通道电压判定"(w1296) -> ()
                  n805 = global write "读配置文件全局2.vi" "保险位置判定"(w1296) -> ()
                  n806 = global write "读配置文件全局2.vi" "二级故障判定"(w1296) -> ()
                  n807 = global write "读配置文件全局2.vi" "三级故障判定"(w1296) -> ()
                  n808 = global write "读配置文件全局2.vi" "电压起始值判定"(w1296) -> ()
                  n809 = global write "读配置文件全局2.vi" "温度起始值判定"(w1296) -> ()
                  n810 = global write "读配置文件全局2.vi" "一级故障判定"(w1296) -> ()
                  n811 = disable-structure shown="禁用" {
                    frame Disabled {
                      n812 = global read "读配置文件全局2.vi" "充电次数时间判定"() -> ()  [unwired: 1 in]
                      n813 = global read "读配置文件全局2.vi" "电池包信息1判定"() -> ()  [unwired: 1 in]
                      n814 = global read "读配置文件全局2.vi" "电池包序号判定"() -> ()  [unwired: 1 in]
                      n815 = global read "读配置文件全局2.vi" "充放电安时判定"() -> ()  [unwired: 1 in]
                      n816 = global read "读配置文件全局2.vi" "车牌号判定"() -> ()  [unwired: 1 in]
                      n817 = global read "读配置文件全局2.vi" "充电参数判定"() -> ()  [unwired: 1 in]
                      n818 = global read "读配置文件全局2.vi" "保险位置判定"() -> ()  [unwired: 1 in]
                    }
                    frame Enabled {
                    }
                  }
                  n819 = property class="Clust (严格)"(reference=w1295, "Value"=T8 {"从板号"=FALSE, "电压起始值"=FALSE, "通道电压数"=FALSE, "保险位置"=FALSE, "温度起始值"=FALSE, "一级故障"=FALSE, "二级故障"=FALSE, "三级故障"=FALSE} ("值")) -> ()  [unwired: 1 in, 2 out]
                }
              }
            }
            frame #1 {
              n820 = call <vilib>:"Open Config Data.vi"("error in (no error)"=w1300, "create file if necessary (T)"=FALSE, "configuration file path"=path "D:/自动测试项目文件/ProjectSetting.ini") -> ("error out"=w1315:errorcluster, "refnum"=w1317:T26)  [unwired: 6 in, 1 out]
              n821 = call <vilib>:"Open Config Data.vi"("error in (no error)"=w1300, "create file if necessary (T)"=FALSE, "configuration file path"=path "D:/BlueWay/BMU从板号.ini") -> ("error out"=w1303:errorcluster, "refnum"=w1301:T26)  [unwired: 6 in, 1 out]
              n822 = call-poly <vilib>:"Read Key.vi"("section"="PROJECT", "error in (no error)"=w1315, "key"="配置文件", "refnum"=w1317) -> ("error out"=w1310:errorcluster, "value"=w1308:string, "refnum out"=w1311:T26)  [unwired: 4 in, 1 out]
              n823 = call <vilib>:"Close Config Data.vi"("error in (no error)"=w1310, "refnum"=w1311) -> ()  [unwired: 8 in, 2 out]
              n824 = call-poly <vilib>:"Read Key.vi"("section"="BMUNO", "error in (no error)"=w1303, "key"="BMUNO", "refnum"=w1301) -> ("error out"=w1306:errorcluster, "value"=w1297:string, "refnum out"=w1305:T26)  [unwired: 4 in, 1 out]
              n825 = call <vilib>:"Close Config Data.vi"("error in (no error)"=w1306, "refnum"=w1305) -> ()  [unwired: 8 in, 2 out]
              n826 = disable-structure shown="禁用" {
                disable-tunnel: w1297 -> [w1328 _]
                frame Disabled {
                  n827 = Decimal String To Number(string=w1328) -> (number=w1327:i32)  [unwired: 2 in, 1 out]
                  n828 = local write "从板号"(w1327) -> ()
                }
                frame Enabled {
                }
              }
              n829 = Build Path(base path=path "D:/自动测试项目文件" ("configuration file path"), name or relative path=w1308) -> (appended path=w1307:path)
              n830 = Strip Path(path=w1307) -> (stripped path=w1318:path, name=w1325:string)
              n831 = Match Pattern(string=w1325, regular expression=".ini" ("正则表达式")) -> (offset past match=w1323:i32)  [unwired: 1 in, 3 out]
              n832 = Not Equal?(x=w1323, y=-1) -> (x != y?=w1319:bool)
              n833 = case shown="真" w1319 {
                tunnel: w1307 -> [_ w1337]
                tunnel: [_ w1346] -> w1320
                frame False {
                }
                frame True {
                  w1349 = "MD5码" ("key")
                  w1350 = "总信息" ("section")
                  n834 = Strip Path(path=w1337) -> (stripped path=w1335:path, name=w1334:string)
                  n835 = Match Pattern(string=w1334, regular expression=".ini" ("正则表达式")) -> (before substring=w1331:string, match substring=w1332:string)  [unwired: 1 in, 2 out]
                  n836 = Concatenate Strings(w1331, "-rc" ("字符串"), w1332) -> (w1330:string)
                  n837 = Build Path(base path=w1335, name or relative path=w1330) -> (appended path=w1336:path)
                  n838 = Copy(10:w1336, 11:w1337) -> (3:w1341:path)  [unwired: 3 in, 2 out]
                  n839 = call <vilib>:"Open Config Data.vi"("create file if necessary (T)"=FALSE, "configuration file path"=w1341) -> ("refnum"=w1352:T26)  [unwired: 7 in, 2 out]
                  n840 = call-poly <vilib>:"Read Key.vi"("section"=w1350, "key"=w1349, "refnum"=w1352) -> ("value"=w1347:string, "refnum out"=w1351:T26)  [unwired: 5 in, 2 out]
                  n841 = call-poly <vilib>:"Write Key.vi"("section"=w1350, "value"=w1349, "key"=w1349, "refnum"=w1351) -> ("error out"=w1345:errorcluster, "found?"=w1344:bool, "refnum out"=w1343:T26)  [unwired: 5 in]
